vi "(SubVI)Scope_Sensor Scale Setting.vi"(7 "error in (no error)":errorcluster caption="에러 입력(에러 없음)") -> (0 "error out":errorcluster caption="에러 출력")   [LabVIEW 2020]
uses:
  Serial/Controls/(Ctrl)Serial_Write Read Option.ctl
  Controls/(Ctrl)Scope_Sensor Scale Setting.ctl
  Controls/(Ctrl)Scope_Sensor Scale Enum.ctl
  Serial/Instance VIs/(SubVI)Serial_Write-Read.vi
panel:
  out "Read Data":u8[](array[numeric])
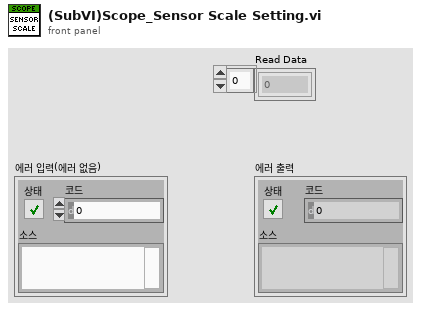
[diagram p1: front panel]
types:
  T1 = typedef "(Ctrl)Scope_Sensor Scale Setting.ctl" = cluster{"Set":bool, "Range":T2}
  T2 = typedef "(Ctrl)Scope_Sensor Scale Enum.ctl" = enum8{"2g", "4g", "8g", "16g"}
  T3 = typedef "(Ctrl)Serial_Write Read Option.ctl" = cluster{"Echo Request":bool, "Header Verification":bool, "Checksum Verification":bool, "User Code Verifiaction":bool}
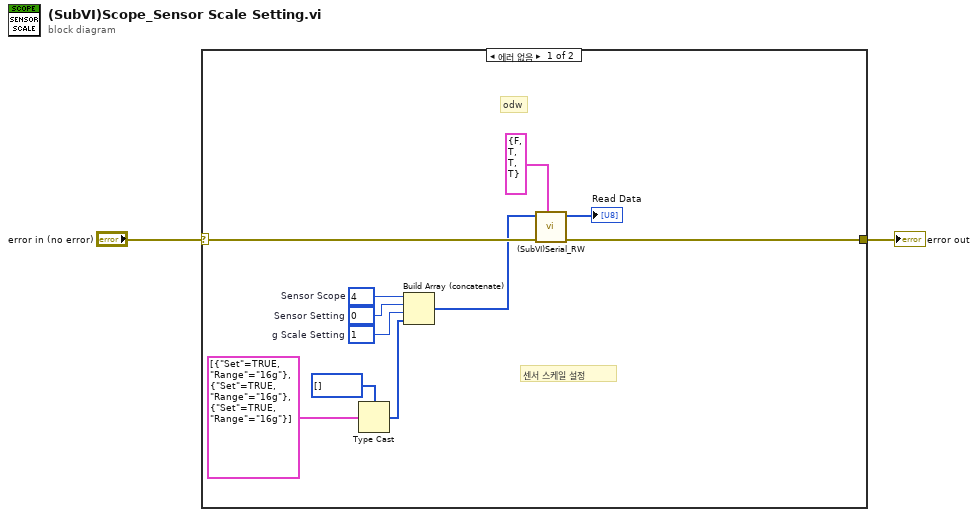
[diagram p0: block diagram]
diagram:
  n1 = case shown="에러 없음" "error in (no error)" {
    selector: "error in (no error)" -> [w11 w14]
    tunnel: [w9 w14] -> w2
    frame No Error {
      w8 = u8 0  # Sensor Setting
      w12 = u8 1  # g Scale Setting
      w13 = u8 4  # Sensor Scope
      # "odw"
      # "센서 스케일 설정"
      n2 = Type Cast(type=u8[] [], x=T1[] [{"Set"=TRUE, "Range"=enum."16g"}, {"Set"=TRUE, "Range"=enum."16g"}, {"Set"=TRUE, "Range"=enum."16g"}] ("배열")) -> (*(type *) &x=w3:u8[])
      n3 = Build Array (concatenate)(w13, w8, w12, w3) -> (w10:u8[])
      n4 = call-poly "(SubVI)Serial_RW.vi"("Option"=T3 {"Echo Request"=FALSE, "Header Verification"=TRUE, "Checksum Verification"=TRUE, "User Code Verifiaction"=TRUE}, "error in (no error)"=w11, "Data to Write"=w10) -> ("error out"=w9:errorcluster, "Read Data"=→"Read Data":u8[])  [unwired: 6 in, 1 out]
    }
    frame Error {
    }
  }
  "error out" <- w2
